vi "datafinder DLL.vi"() -> ()   [LabVIEW 2011]
panel:
  out "Array 3":string[][](array[string])
  out "Array 2":string[][](array[string])
  out "Array 4":i32[](array[numeric])
  out "error out":errorcluster
  out "IsIncomplete":i32
  out "Array":string[](array[string])
  out "Indexed properties":T1(array[cluster])
  in  "Value":string[](array[string])=["*jamestest*", "s parameter"]
  in  "Type":string[](array[string])=["file", "tdm_channelgroup"]
  in  "Property":string[](array[string])=["Filename", "Test_Type"]
  in  "Operator":string[](array[string])=["=", "="]
  in  "Logic":string="C1 AND C2"
  in  "SUSIResultsDisplay":refnum<k7>(container)
  in  "SUSIQueryForm":refnum<k7>(container)
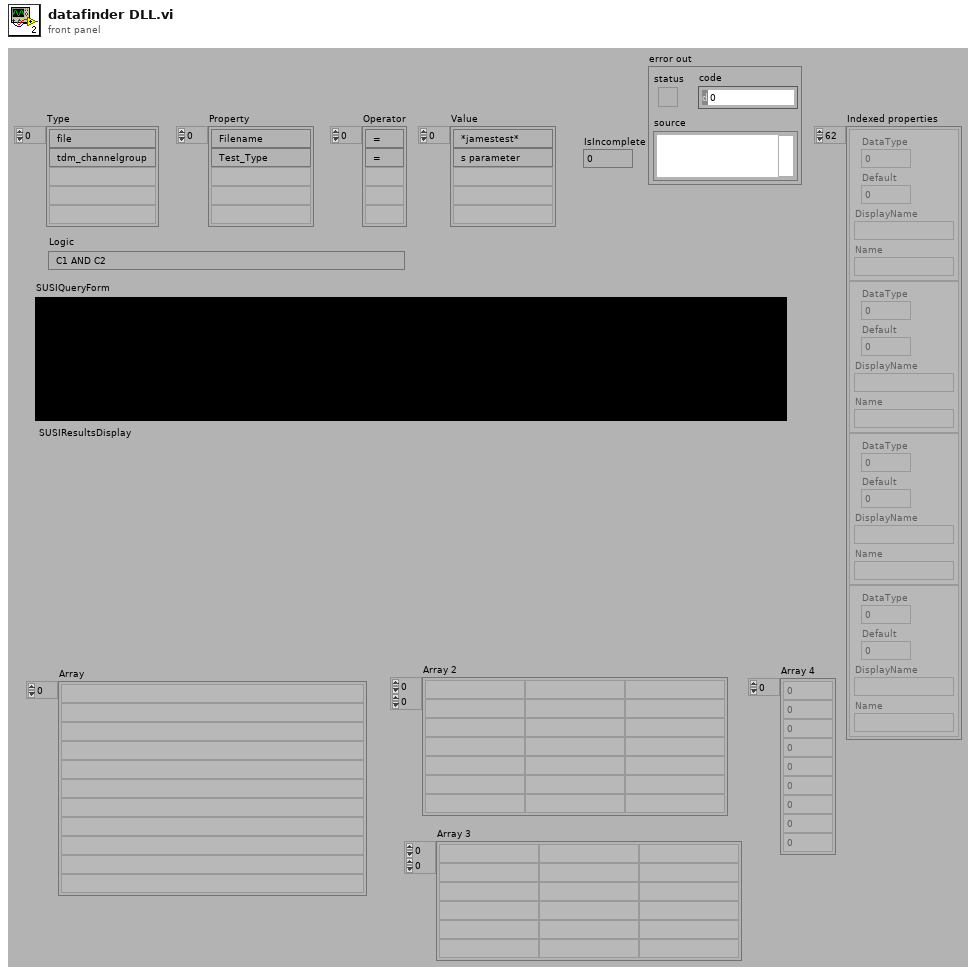
[diagram p1: front panel]
types:
  T1 = cluster{"DataType":i32, "Default":i32, "DisplayName":string, "Name":string}[]
  T2 = cluster{"DataType":i32, "Default":i32, "DisplayName":string, "Name":string}
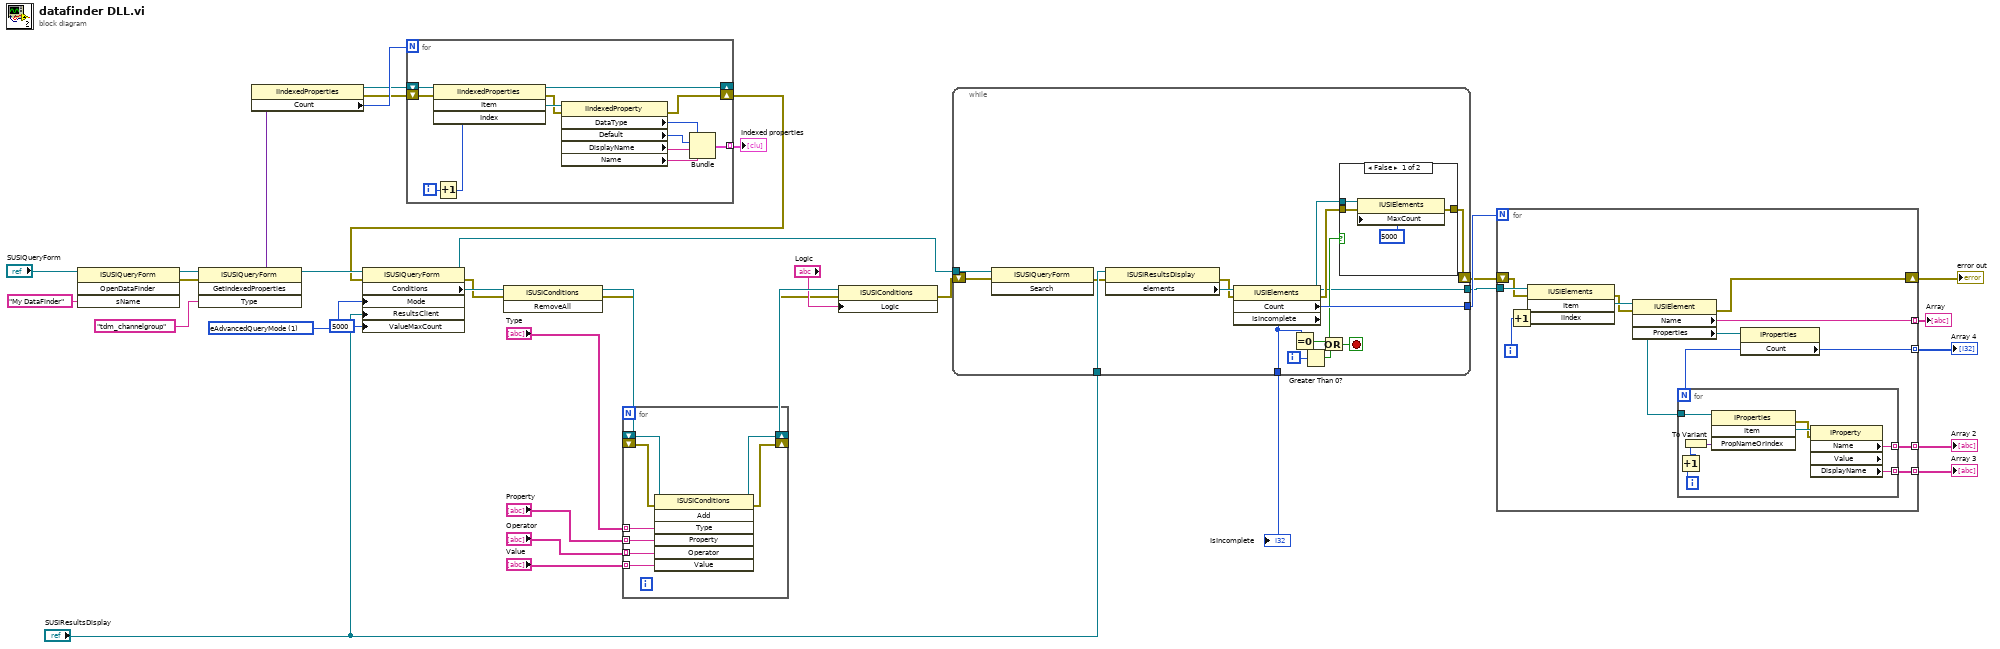
[diagram p0: block diagram]
diagram:
  w22 = 1 items=["eAdvancedQueryMode"=1, "eQuickQueryMode"=2] ("Mode")
  n1 = invoke class="ISUSIQueryForm" method="OpenDataFinder"(reference="SUSIQueryForm", "sName"="My DataFinder") -> (reference out=w21:refnum<k7>, error out=w20:errorcluster)  [unwired: 2 in, 2 out]
  n2 = invoke class="ISUSIQueryForm" method="GetIndexedProperties"(reference=w21, error in=w20, "Type"="tdm_channelgroup") -> (reference out=w19:refnum<k7>, "GetIndexedProperties"=w17:variant)  [unwired: 1 in, 2 out]
  n3 = property class="IIndexedProperties"(reference=w17) -> (reference out=w15:refnum<k7>, error out=w14:errorcluster, "Count"=w16:i32)  [unwired: 1 in]
  n4 = for {
    N: w16 -> [_]
    shift-right: [w49] -> _
    shift-left: w15 -> [w50]
    shift-right: [w39] -> w13
    shift-left: w14 -> [w48]
    tunnel: [w38] -> w12 mode=indexing
    i -> [w46]
    n5 = Increment(x=w46) -> (x+1=w45:i32)
    n6 = invoke class="IIndexedProperties" method="Item"(reference=w50, error in=w48, "Index"=w45) -> (reference out=w49:refnum<k7>, error out=w40:errorcluster, "Item"=w47:refnum<k7>)  [unwired: 1 in, 1 out]
    n7 = property class="IIndexedProperty"(reference=w47, error in=w40) -> (error out=w39:errorcluster, "DataType"=w41:i32, "Default"=w42:i32, "DisplayName"=w43:string, "Name"=w44:string)  [unwired: 1 out]
    n8 = Bundle("DataType"=w41, "Default"=w42, "DisplayName"=w43, "Name"=w44) -> (w38:T2)  [unwired: 1 out]
  }
  "Indexed properties" <- w12
  n9 = property class="ISUSIQueryForm"(reference=w19, error in=w13, "Mode"=w22, "ResultsClient"="SUSIResultsDisplay", "ValueMaxCount"=5000) -> (reference out=w24:refnum<k7>, error out=w27:errorcluster, "Conditions"=w35:refnum<k7>)
  n10 = invoke class="ISUSIConditions" method="RemoveAll"(reference=w35, error in=w27) -> (reference out=w30:refnum<k7>, error out=w26:errorcluster)  [unwired: 1 in, 1 out]
  n11 = for {
    tunnel: "Type" -> [w58] mode=indexing
    tunnel: "Property" -> [w57] mode=indexing
    tunnel: "Operator" -> [w56] mode=indexing
    tunnel: "Value" -> [w55] mode=indexing
    shift-right: [w53] -> w29
    shift-left: w30 -> [w54]
    shift-right: [w51] -> w25
    shift-left: w26 -> [w52]
    n12 = invoke class="ISUSIConditions" method="Add"(reference=w54, error in=w52, "Type"=w58, "Property"=w57, "Operator"=w56, "Value"=w55) -> (reference out=w53:refnum<k7>, error out=w51:errorcluster)  [unwired: 1 in, 5 out]
  }
  n13 = property class="ISUSIConditions"(reference=w29, error in=w25, "Logic"="Logic") -> (error out=w23:errorcluster)  [unwired: 1 out]
  n14 = while {
    tunnel: w24 -> [w73]
    tunnel: "SUSIResultsDisplay" -> [w71]
    tunnel: [w67] -> w11
    tunnel: [w59] -> w10
    tunnel: [w66] -> w7
    shift-right: [w62] -> w5
    shift-left: w23 -> [w72]
    i -> [w61]
    stop <- w65 stop-if-true
    n15 = invoke class="ISUSIQueryForm" method="Search"(reference=w73, error in=w72) -> (error out=w70:errorcluster)  [unwired: 1 in, 2 out]
    n16 = property class="ISUSIResultsDisplay"(reference=w71, error in=w70) -> (error out=w68:errorcluster, "elements"=w69:refnum<k7>)  [unwired: 1 out]
    n17 = property class="IUSIElements"(reference=w69, error in=w68) -> (reference out=w59:refnum<k7>, error out=w63:errorcluster, "Count"=w67:i32, "IsIncomplete"=w66:i32)
    n18 = Equal To 0?(x=w66) -> (x = 0?=w64:bool)
    n19 = Greater Than 0?(x=w61) -> (x > 0?=w60:bool)
    n20 = Or(x=w64, y=w60) -> (x .or. y?=w65:bool)
    n21 = case shown="False" w64 {
      tunnel: w63 -> [w77 w78]
      tunnel: [w76 w78] -> w62
      tunnel: w59 -> [w74 _]
      frame False {
        n22 = property class="IUSIElements"(reference=w74, error in=w77, "MaxCount"=5000 ("ValueMaxCount")) -> (error out=w76:errorcluster)  [unwired: 1 out]
      }
      frame True {
      }
    }
  }
  "IsIncomplete" <- w7
  n23 = for {
    N: w11 -> [_]
    tunnel: w10 -> [w90]
    tunnel: [w88] -> w9 mode=indexing
    tunnel: [w85] -> w2 mode=indexing
    tunnel: [w84] -> w1 mode=indexing
    shift-right: [w81] -> w4
    shift-left: w5 -> [w82]
    tunnel: [w79] -> w3 mode=indexing
    i -> [w87]
    n24 = Increment(x=w87) -> (x+1=w86:i32)
    n25 = invoke class="IUSIElements" method="Item"(reference=w90, error in=w82, "iIndex"=w86) -> (error out=w83:errorcluster, "Item"=w89:refnum<k7>)  [unwired: 1 in, 2 out]
    n26 = property class="IUSIElement"(reference=w89, error in=w83) -> (error out=w81:errorcluster, "Name"=w88:string, "Properties"=w80:refnum<k7>)  [unwired: 1 out]
    n27 = property class="IProperties"(reference=w80) -> ("Count"=w79:i32)  [unwired: 1 in, 2 out]
    n28 = for {
      N: w79 -> [_]
      tunnel: [w97] -> w85 mode=indexing
      tunnel: [w96] -> w84 mode=indexing
      tunnel: w80 -> [w93]
      i -> [w92]
      n29 = Increment(x=w92) -> (x+1=w91:i32)
      n30 = To Variant(anything=w91) -> (Variant=w95:variant)
      n31 = invoke class="IProperties" method="Item"(reference=w93, "PropNameOrIndex"=w95) -> (error out=w94:errorcluster, "Item"=w98:refnum<k7>)  [unwired: 2 in, 2 out]
      n32 = property class="IProperty" props=["Name", "Value", "DisplayName"](reference=w98, error in=w94) -> ("Name"=w97:string, "DisplayName"=w96:string)  [unwired: 3 out]
    }
  }
  "Array" <- w9
  "error out" <- w4
  "Array 4" <- w3
  "Array 2" <- w2
  "Array 3" <- w1
